vi "Reset.vi"(8 "error in (no error)":errorcluster, 11 "Serial Port in":refnum<visa-resource-name>) -> (0 "error out":errorcluster, 3 "Serial Port out":refnum<visa-resource-name>)   [LabVIEW 2015, in "Chemyx_Syringe_Pump_driver.lvlib"]
doc: "Restarts the pump."
uses:
  Chemyx_Syringe_Pump_driver.lvlib
panel:
  # "Restarts the pump."
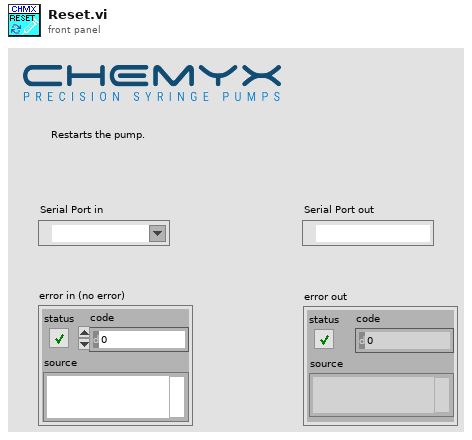
[diagram p1: front panel]
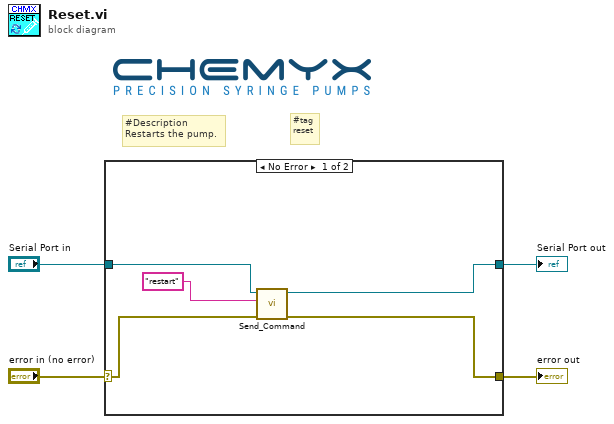
[diagram p0: block diagram]
diagram:
  # "#tag\nreset"
  # "#Description\nRestarts the pump."
  n1 = case shown="No Error" "error in (no error)" {
    selector: "error in (no error)" -> [w8 w11]
    tunnel: "Serial Port in" -> [w9 w10]
    tunnel: [w6 w11] -> w2
    tunnel: [w5 w10] -> w1
    frame No Error {
      n2 = call "Send_Command.vi"("error in (no error)"=w8, "write buffer"="restart", "Serial Port in"=w9) -> ("error out"=w6:errorcluster, "VISA Refnum out"=w5:refnum<visa-resource-name>)  [unwired: 6 in, 1 out]
    }
    frame Error {
    }
  }
  "error out" <- w2
  "Serial Port out" <- w1
